vi "Is Fixed-Size.vi"(10 "Data Type":T1) -> (2 "Is Fixed-Size":bool)   [LabVIEW 2017, in "Composition.lvlib"]
doc: "Returns true if the provided type is fixed-size."
uses:
  Composition.lvlib
  Data Type.ctl
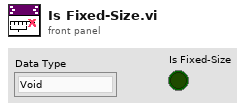
[diagram p1: front panel]
types:
  T1 = typedef "Composition.lvlib/Data Type.ctl" = enum16{"Void", "I8", "I16", "I32", "I64", "U8", "U16", "U32", "U64", "SGL", "DBL", "EXT", "CSG", "CDB", "CXT", "0x0F", "0x10", "0x11", "0x12", "0x13", "0x14", "Enum U8", "Enum U16", "Enum U32", "0x18", "SGL Physical", "DBL Physical", "EXT Physical", "CSG Physical", "CDB Physical", "CXT Physical", "0x1F", "Boolean U16", "Boolean U8", "0x22", "0x23", "0x24", "0x25", "0x26", "0x27", "0x28", "0x29", "0x2A", "0x2B", "0x2C", "0x2D", "0x2E", "0x2F", "String", "0x31", "Path", "Picture", "CString", "PString", "0x36", "Tag", "0x38", "0x39", "0x3A", "0x3B", "0x3C", "0x3D", "0x3E", "SubString", "Array", "Array Data Ptr", "0x42", "0x43", "0x44", "0x45", "0x46", "0x47", "0x48", "0x49", "0x4A", "0x4B", "0x4C", "0x4D", "0x4E", "SubArray", "Cluster", "0x51", "0x52", "Variant", "Waveform", "0x55", "0x56", "0x57", "0x58", "0x59", "0x5A", "0x5B", "0x5C", "0x5D", "CFX", "FXP", "Block", "Type Block", "Void Block", "Aligned Block", "Repeated Block", "Alignment Marker", "0x66", "0x67", "0x68", "0x69", "0x6A", "0x6B", "0x6C", "0x6D", "0x6E", "0x6F", "Refnum", "0x71", "0x72", "Set Collection", "Map Collection", "0x75", "0x76", "0x77", "0x78", "0x79", "0x7A", "0x7B", "0x7C", "0x7D", "0x7E", "0x7F", "Ptr", "0x81", "0x82", "Ptr to", "EXT Data", "0x85", "0x86", "0x87", "0x88", "0x89", "0x8A", "0x8B", "0x8C", "0x8D", "0x8E", "0x8F", "0x90", "0x91", "0x92", "0x93", "0x94", "0x95", "0x96", "0x97", "0x98", "0x99", "0x9A", "0x9B", "0x9C", "0x9D", "0x9E", "0x9F", "Array Interface", "Interface to Data", "0xA2", "0xA3", "0xA4", "0xA5", "0xA6", "0xA7", "0xA8", "0xA9", "0xAA", "0xAB", "0xAC", "0xAD", "0xAE", "0xAF", "0xB0", "0xB1", "0xB2", "0xB3", "0xB4", "0xB5", "0xB6", "0xB7", "0xB8", "0xB9", "0xBA", "0xBB", "0xBC", "0xBD", "0xBE", "0xBF", "0xC0", "0xC1", "0xC2", "0xC3", "0xC4", "0xC5", "0xC6", "0xC7", "0xC8", "0xC9", "0xCA", "0xCB", "0xCC", "0xCD", "0xCE", "0xCF", "0xD0", "0xD1", "0xD2", "0xD3", "0xD4", "0xD5", "0xD6", "0xD7", "0xD8", "0xD9", "0xDA", "0xDB", "0xDC", "0xDD", "0xDE", "0xDF", "0xE0", "0xE1", "0xE2", "0xE3", "0xE4", "0xE5", "0xE6", "0xE7", "0xE8", "0xE9", "0xEA", "0xEB", "0xEC", "0xED", "0xEE", "0xEF", "Function", "TypeDef", "PolyVI", "0xF3", "0xF4", "0xF5", "0xF6", "0xF7", "0xF8", "0xF9", "0xFA", "0xFB", "0xFC", "0xFD", "0xFE", "0xFF"}
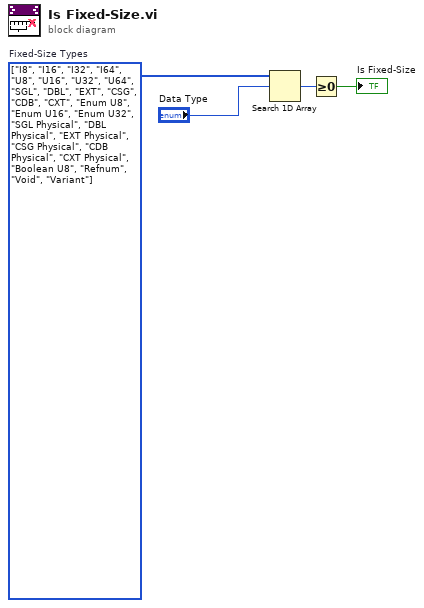
[diagram p0: block diagram]
diagram:
  w4 = T1[] [enum."I8", enum."I16", enum."I32", enum."I64", enum."U8", enum."U16", enum."U32", enum."U64", enum."SGL", enum."DBL", enum."EXT", enum."CSG", enum."CDB", enum."CXT", enum."Enum U8", enum."Enum U16", enum."Enum U32", enum."SGL Physical", enum."DBL Physical", enum."EXT Physical", enum."CSG Physical", enum."CDB Physical", enum."CXT Physical", enum."Boolean U8", enum."Refnum", enum."Void", enum."Variant"] items=["Void", "I8", "I16", "I32", "I64", "U8", "U16", "U32", "U64", "SGL", "DBL", "EXT", "CSG", "CDB", "CXT", "0x0F", "0x10", "0x11", "0x12", "0x13", "0x14", "Enum U8", "Enum U16", "Enum U32", "0x18", "SGL Physical", "DBL Physical", "EXT Physical", "CSG Physical", "CDB Physical", "CXT Physical", "0x1F", "Boolean U16", "Boolean U8", "0x22", "0x23", "0x24", "0x25", "0x26", "0x27", "0x28", "0x29", "0x2A", "0x2B", "0x2C", "0x2D", "0x2E", "0x2F", "String", "0x31", "Path", "Picture", "CString", "PString", "0x36", "Tag", "0x38", "0x39", "0x3A", "0x3B", "0x3C", "0x3D", "0x3E", "SubString", "Array", "Array Data Ptr", "0x42", "0x43", "0x44", "0x45", "0x46", "0x47", "0x48", "0x49", "0x4A", "0x4B", "0x4C", "0x4D", "0x4E", "SubArray", "Cluster", "0x51", "0x52", "Variant", "Waveform", "0x55", "0x56", "0x57", "0x58", "0x59", "0x5A", "0x5B", "0x5C", "0x5D", "CFX", "FXP", "Block", "Type Block", "Void Block", "Aligned Block", "Repeated Block", "Alignment Marker", "0x66", "0x67", "0x68", "0x69", "0x6A", "0x6B", "0x6C", "0x6D", "0x6E", "0x6F", "Refnum", "0x71", "0x72", "Set Collection", "Map Collection", "0x75", "0x76", "0x77", "0x78", "0x79", "0x7A", "0x7B", "0x7C", "0x7D", "0x7E", "0x7F", "Ptr", "0x81", "0x82", "Ptr to", "EXT Data", "0x85", "0x86", "0x87", "0x88", "0x89", "0x8A", "0x8B", "0x8C", "0x8D", "0x8E", "0x8F", "0x90", "0x91", "0x92", "0x93", "0x94", "0x95", "0x96", "0x97", "0x98", "0x99", "0x9A", "0x9B", "0x9C", "0x9D", "0x9E", "0x9F", "Array Interface", "Interface to Data", "0xA2", "0xA3", "0xA4", "0xA5", "0xA6", "0xA7", "0xA8", "0xA9", "0xAA", "0xAB", "0xAC", "0xAD", "0xAE", "0xAF", "0xB0", "0xB1", "0xB2", "0xB3", "0xB4", "0xB5", "0xB6", "0xB7", "0xB8", "0xB9", "0xBA", "0xBB", "0xBC", "0xBD", "0xBE", "0xBF", "0xC0", "0xC1", "0xC2", "0xC3", "0xC4", "0xC5", "0xC6", "0xC7", "0xC8", "0xC9", "0xCA", "0xCB", "0xCC", "0xCD", "0xCE", "0xCF", "0xD0", "0xD1", "0xD2", "0xD3", "0xD4", "0xD5", "0xD6", "0xD7", "0xD8", "0xD9", "0xDA", "0xDB", "0xDC", "0xDD", "0xDE", "0xDF", "0xE0", "0xE1", "0xE2", "0xE3", "0xE4", "0xE5", "0xE6", "0xE7", "0xE8", "0xE9", "0xEA", "0xEB", "0xEC", "0xED", "0xEE", "0xEF", "Function", "TypeDef", "PolyVI", "0xF3", "0xF4", "0xF5", "0xF6", "0xF7", "0xF8", "0xF9", "0xFA", "0xFB", "0xFC", "0xFD", "0xFE", "0xFF"]  # Fixed-Size Types
  n1 = Search 1D Array(1D array=w4, element="Data Type") -> (index of element=w2:i32)  [unwired: 1 in]
  n2 = Greater Or Equal To 0?(x=w2) -> (x >= 0?=→"Is Fixed-Size":bool)
